vi "UTILITY Remove Zeros.vi"(11 "Array in":dbl[](array[numeric])) -> (3 "Array out":dbl[](array[numeric]))   [LabVIEW 2018]
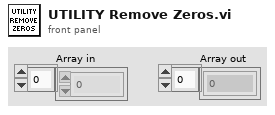
[diagram p1: front panel]
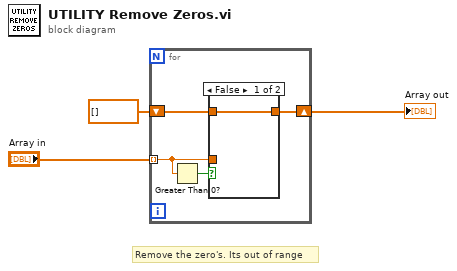
[diagram p0: block diagram]
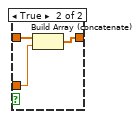
[diagram p2: hidden frame]
diagram:
  # "Remove the zero's. Its out of range"
  n1 = for {
    tunnel: "Array in" -> [w5] mode=indexing
    shift-right: [w4] -> w3
    shift-left: dbl[] [] -> [w6]
    n2 = Greater Than 0?(x=w5) -> (x > 0?=w7:bool)
    n3 = case shown="False" w7 {
      tunnel: w6 -> [w8 w11]
      tunnel: w5 -> [_ w10]
      tunnel: [w8 w9] -> w4
      frame False {
      }
      frame True {
        n4 = Build Array (concatenate)(w11, w10) -> (w9:dbl[])
      }
    }
  }
  "Array out" <- w3
